vi "Input Test.vi"() -> ()   [LabVIEW 2016]
uses:
  <vilib>/Rock Robotics/WPI/Joystick/WPI_JoystickDeviceEnum.ctl
panel:
  in  "stop":bool
  out "Throttle":u8(slide) scale=0.0..100.0
  out "Y-Axis":u8(slide) scale=0.0..100.0
  out "X-Axis":u8(slide) scale=0.0..100.0
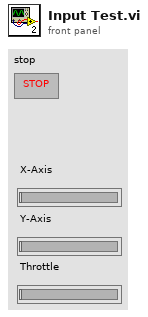
[diagram p1: front panel]
types:
  T1 = typedef "WPI_JoystickDeviceEnum.ctl" = enum16{"USB 0", "USB 1", "USB 2", "USB 3", "USB 4", "USB 5"}
  T2 = typedef "WPI_JoystickDevRef.ctl" = cluster{"Device":T1}
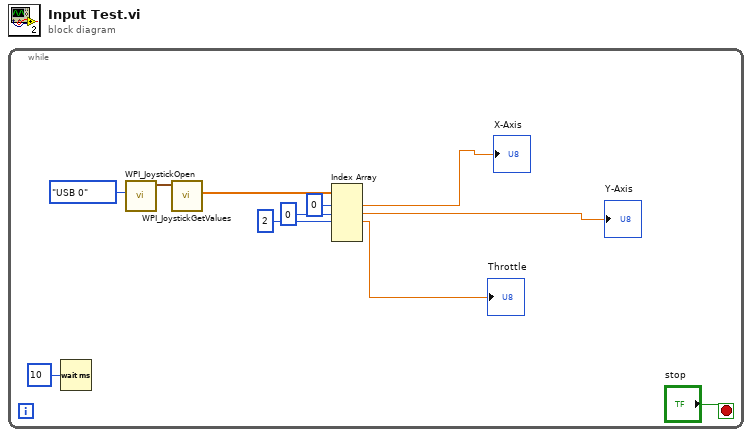
[diagram p0: block diagram]
diagram:
  n1 = while {
    stop <- "stop" stop-if-true
    n2 = Wait (ms)(milliseconds to wait=u32 10) -> ()  [unwired: 1 out]
    n3 = call <vilib>:"WPI_JoystickOpen.vi"("JoystickDevice"=WPI_JoystickDeviceEnum."USB 0") -> ("JoystickDevRef"=w10:T2)  [unwired: 10 in]
    n4 = call <vilib>:"WPI_JoystickGetValues.vi"("JoystickDevRef"=w10) -> ("Axes"=w9:dbl[])  [unwired: 6 in, 4 out]
    n5 = Index Array(array=w9, index #1=0 ("index"), index #2=0 ("index"), index #3=2 ("index")) -> (element #1=→"X-Axis":dbl, element #2=→"Y-Axis":dbl, element #3=→"Throttle":dbl)  [unwired: 2 in, 2 out]
  }
